vi "StartVideo PictureBox.vi"(0 "VLC Variables In":T1, 1 "PictureBox":refnum<k24>(container), 9 "Media Source":string="dshow://", 11 "error in (no error)":errorcluster) -> (4 "VLC Variables Out":T1, 15 "error out":errorcluster)   [LabVIEW 2012]
doc: "Set up all option to start streaming video from the webcam"
uses:
  Controls-Webcam/VLC Var.ctl
  System.Windows.Forms
panel:
  in  "Script":string
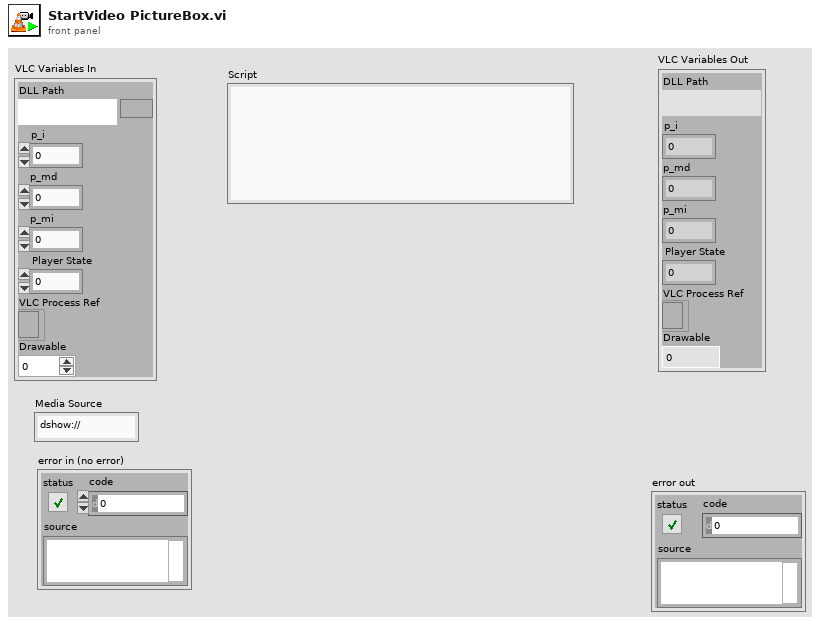
[diagram p1: front panel]
types:
  T1 = typedef "VLC Var.ctl" = cluster{"DLL Path":path, "p_i":i32, "p_md":i32, "p_mi":i32, "Player State":i32, "VLC Process Ref":refnum<k24>, "Drawable":i32}
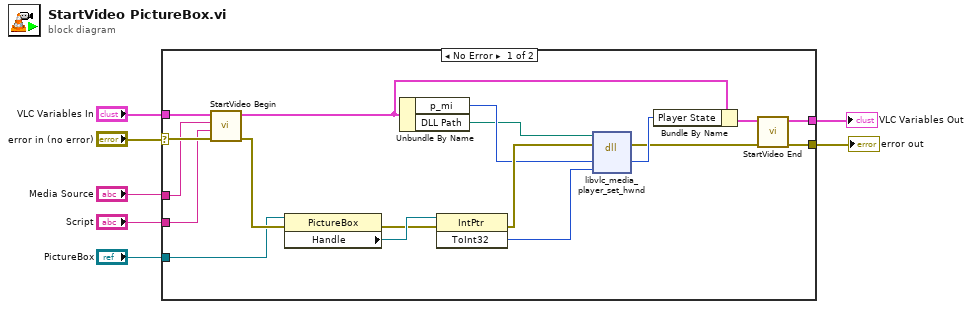
[diagram p0: block diagram]
diagram:
  n1 = case shown="No Error" "error in (no error)" {
    selector: "error in (no error)" -> [w19 w26]
    tunnel: [w16 w27] -> w7
    tunnel: [w15 w26] -> w6
    tunnel: "Script" -> [w9 _]
    tunnel: "VLC Variables In" -> [w8 w27]
    tunnel: "PictureBox" -> [w11 _]
    tunnel: "Media Source" -> [w10 _]
    frame No Error {
      n2 = call "StartVideo Begin.vi"("error in (no error)"=w19, "Script"=w9, "Media Source"=w10, "VLC Variables In in"=w8) -> ("error out"=w20:errorcluster, "VLC Variables In out"=w18:T1)  [unwired: 6 in]
      n3 = property class="PictureBox"(reference=w11, error in=w20) -> (error out=w23:errorcluster, "Handle"=w24:refnum<k24>)  [unwired: 1 out]
      n4 = Unbundle By Name(w18) -> ("p_mi"=w17:i32, "DLL Path"=w12:path)
      n5 = invoke class="IntPtr" method="ToInt32"(reference=w24, error in=w23) -> (error out=w21:errorcluster, "ToInt32"=w22:i32)  [unwired: 1 in, 1 out]
      n6 = dll-call lib="C:/Program Files (x86)/VideoLAN/VLC/libvlc.dll" fn="libvlc_media_player_set_hwnd"(path in=w12, error in=w21, "p_mi"=w17, "handle"=w22) -> (error out=w13:errorcluster, "p_mi"=w25:i32)  [unwired: 3 in, 1 out]
      n7 = Bundle By Name(cluster=w18, "Player State"=w25) -> (w14:T1)
      n8 = call "StartVideo End.vi"("error in (no error)"=w13, "VLC Variables In in"=w14) -> ("error out"=w15:errorcluster, "VLC Variables In out"=w16:T1)  [unwired: 8 in]
    }
    frame Error {
    }
  }
  "error out" <- w6
  "VLC Variables Out" <- w7
